vi "Global Variable Application VI.vi"() -> ()   [LabVIEW 2016]
uses:
  Global Variable Control (Front Panel Design of Global Variable).vi
panel:
  out "Waveform Chart":dbl(graph)
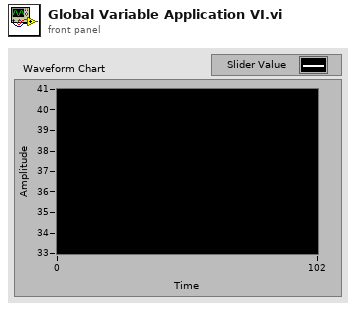
[diagram p1: front panel]
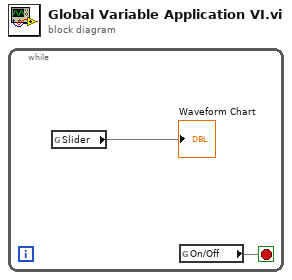
[diagram p0: block diagram]
diagram:
  n1 = while {
    stop <- w1 stop-if-true
    n2 = global read "Global Variable Control (Front Panel Design of Global Variable).vi" "Slider"() -> (→"Waveform Chart")
    n3 = global read "Global Variable Control (Front Panel Design of Global Variable).vi" "On/Off"() -> (w1)
  }
